vi "FileRenamer.vi"() -> ()   [LabVIEW 2018]
uses:
  <vilib>/Utility/file.llb/Read From Spreadsheet File (string).vi
  <vilib>/Utility/file.llb/Write To Spreadsheet File (string).vi
panel:
  in  "replace string (\"\")":string="AV524B001Z"
  in  "search string":string="AV524B"
  in  "path":path
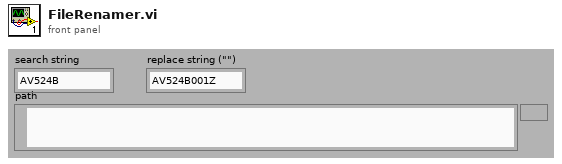
[diagram p1: front panel]
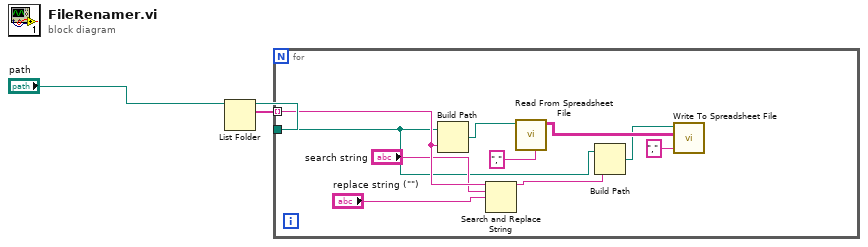
[diagram p0: block diagram]
diagram:
  n1 = List Folder(path="path") -> (path out=w1:path, filenames=w2:string[])  [unwired: 3 in, 2 out]
  n2 = for {
    tunnel: w2 -> [w12] mode=indexing
    tunnel: w1 -> [w5]
    n3 = Build Path(base path=w5, name or relative path=w12) -> (appended path=w13:path)
    n4 = Search and Replace String(input string=w12, search string="search string", replace string="replace string (\"\")") -> (result string=w4:string)  [unwired: 5 in, 3 out]
    n5 = call-poly <vilib>:"Read From Spreadsheet File.vi"("delimiter (\\t)"="," ("delimiter (\\t)"), "file path (dialog if empty)"=w13) -> ("all rows"=w8:string[][])  [unwired: 5 in, 4 out]
    n6 = Build Path(base path=w5, name or relative path=w4) -> (appended path=w6:path)
    n7 = call-poly <vilib>:"Write To Spreadsheet File.vi"("delimiter (\\t)"="," ("delimiter (\\t)"), "2D data"=w8, "file path (dialog if empty)"=w6) -> ()  [unwired: 5 in, 1 out]
  }
